vi "Deform_Mirror_DUAL_AE_V2.vi"(0 "Refnum In":refnum<k7>, 1 "Action":T1, 5 "IDs In":i32[](array[numeric]), 7 "Flat Files In":dbl[][](array[numeric]), 9 "Multi Map Data In":i32[](array[numeric]), 11 "Mode Matrix":dbl[][](array[numeric])) -> (4 "Refnum Out":refnum<k7>, 6 "IDs Out":i32[](array[numeric]), 8 "Flat Files Out":dbl[][](array[numeric]), 10 "Multi Map Data Out":i32[](array[numeric]), 15 "Mode Matrix Out":dbl[][](array[numeric]))   [LabVIEW 2014]
uses:
  Controls/Standard Action.ctl
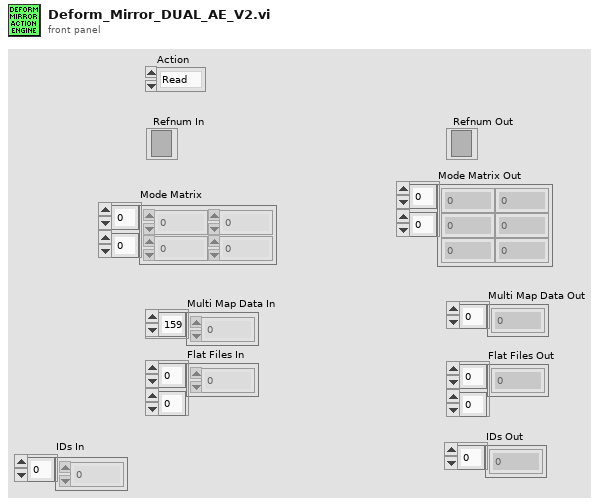
[diagram p1: front panel]
types:
  T1 = typedef "Standard Action.ctl" = enum16{"Read", "Write"}
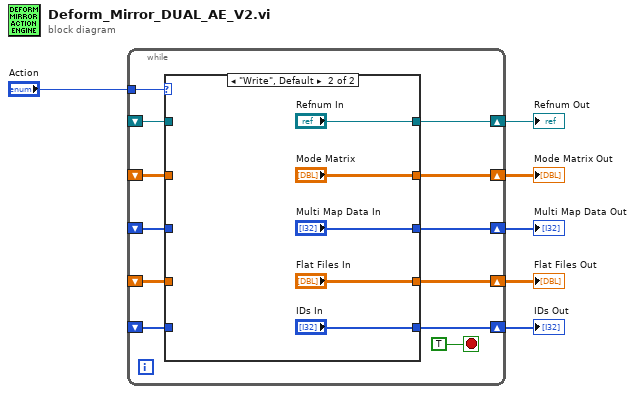
[diagram p0: block diagram]
diagram:
  n1 = while {
    tunnel: "Action" -> [w17]
    shift-right: [w10] -> w2
    shift-left: _ -> [w16]
    shift-right: [w9] -> w1
    shift-left: _ -> [w15]
    shift-right: [w14] -> w5
    shift-left: _ -> [w13]
    shift-right: [w12] -> w3
    shift-left: _ -> [w11]
    shift-right: [w8] -> w4
    shift-left: _ -> [w7]
    stop <- TRUE stop-if-true
    n2 = case shown="\"Write\", Default" w17 {
      tunnel: w16 -> [w21 _]
      tunnel: w15 -> [w20 _]
      tunnel: [w23 "Mode Matrix"] -> w14
      tunnel: w13 -> [w23 _]
      tunnel: [w22 "Multi Map Data In"] -> w12
      tunnel: w11 -> [w22 _]
      tunnel: [w21 "Flat Files In"] -> w10
      tunnel: [w20 "IDs In"] -> w9
      tunnel: [w19 "Refnum In"] -> w8
      tunnel: w7 -> [w19 _]
      frame "Read" {
      }
      frame "Write", Default {
      }
    }
  }
  "Flat Files Out" <- w2
  "Multi Map Data Out" <- w3
  "Refnum Out" <- w4
  "Mode Matrix Out" <- w5
  "IDs Out" <- w1
